vi "Read configuration.vi"(8 "error in":errorcluster, 11 "Sequencer Module editor node in":refnum<class "Sequencer Module editor node.lvclass">) -> (0 "error out":errorcluster, 2 "configuration":refnum<class "NISE_CEF_serializable configuration.lvclass">, 3 "Sequencer Module editor node out":refnum<class "Sequencer Module editor node.lvclass">)   [LabVIEW 2015, in "Sequencer Module editor node.lvclass"]
uses:
  Sequencer Module editor node.lvclass
  <vilib>/NI/Configuration Framework/serializable configuration/NISE_CEF_serializable configuration.lvclass
  Sequencer Module editor node.lvclass/Sequencer Module editor node.ctl
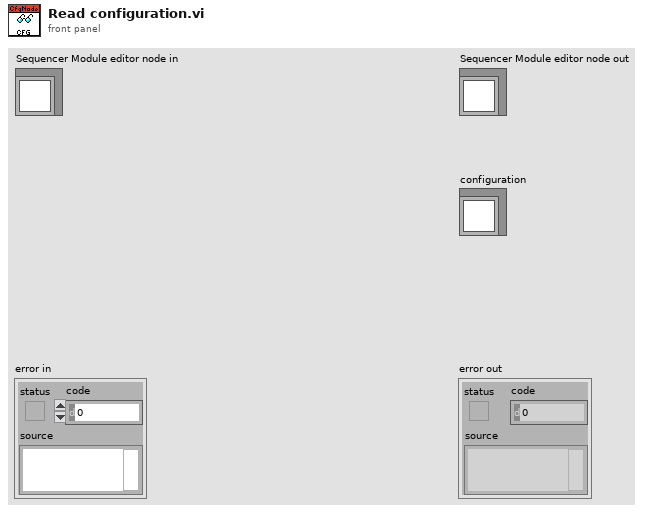
[diagram p1: front panel]
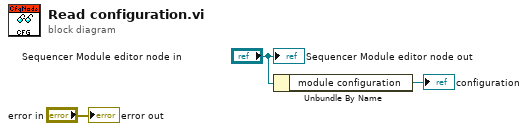
[diagram p0: block diagram]
diagram:
  n1 = Unbundle By Name("Sequencer Module editor node in") -> ("module configuration"=→"configuration":refnum<class "Sequencer Module configuration.lvclass">)
  "error out" <- "error in"
  "Sequencer Module editor node out" <- "Sequencer Module editor node in"
